vi "Main.vi"() -> ()   [LabVIEW 2021]
doc: "Use this template to build a simple state machine design pattern. Each state executes code and determines which state to transition to."
uses:
  controls/State.ctl
  controls/Data.ctl
  vmmultmso/vmmultmso.lvlib
panel:
  out "Device is OK?":bool
  out "Sample Rate":dbl
  out "Device ID":dbl
  out "CH2 Min":dbl
  out "CH2 Max":dbl
  out "CH2 Vpp":dbl
  out "CH2 Frequency":dbl
  out "CH1 Frequency":dbl
  out "CH1 Vpp":dbl
  out "CH1 Max":dbl
  out "CH1 Min":dbl
  out "IO Read Return":u32 format="%x"
  out "IO4":bool
  out "IO0":bool
  out "Is IO Ready?":bool
  in  "DDS2 Amplitude":dbl=2000.0
  in  "DDS2 Bias":dbl
  in  "DDS2 Freq":dbl=1000.0
  in  "DDS2 Wave Style":u16(ring) items=["Sine", "Square", "Ramp"]
  in  "DDS1 Amplitude":dbl=2000.0
  in  "DDS1 Bias":dbl
  in  "DDS1 Freq":dbl=1000.0
  in  "DDS1 Wave Style":u16(ring) items=["Sine", "Square", "Ramp"]
  out "Is Data Ready？":bool
  out "ReadVoltageData Return":u32
  out "Voltage Wave":dbl[][](graph)
  out "Capture Return":i32
  out "Support Samples":u32[](array[numeric])
  in  "Exit":bool
  # "DDS1"
  # "DDS2"
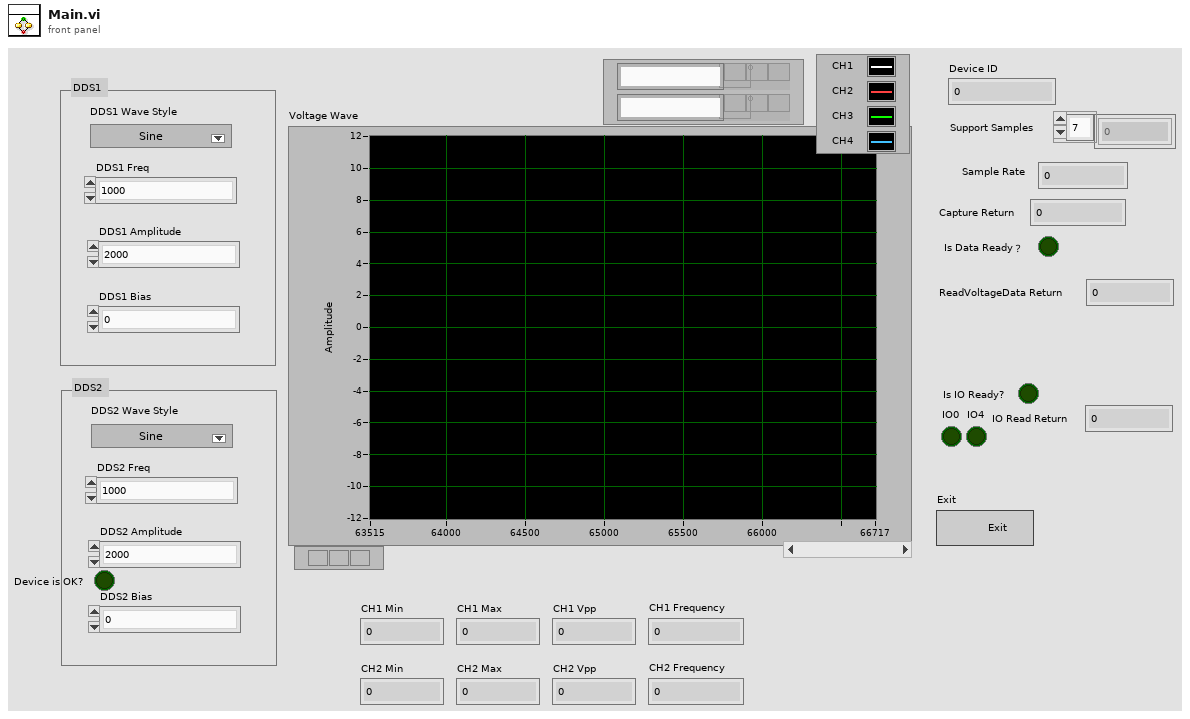
[diagram p1: front panel]
types:
  T1 = typedef "Data.ctl" = cluster{"Boolean <Is Exit>":bool, "String <Replace Me>":string, "Captue Length":dbl, "Device ID":dbl}
  T2 = typedef "State.ctl" = enum16{"Initialize", "Wait for UsbIn", "Init Osc and Dds", "Wait for Event", "Capture", "Read Voltage", "Read IO", "Exit"}
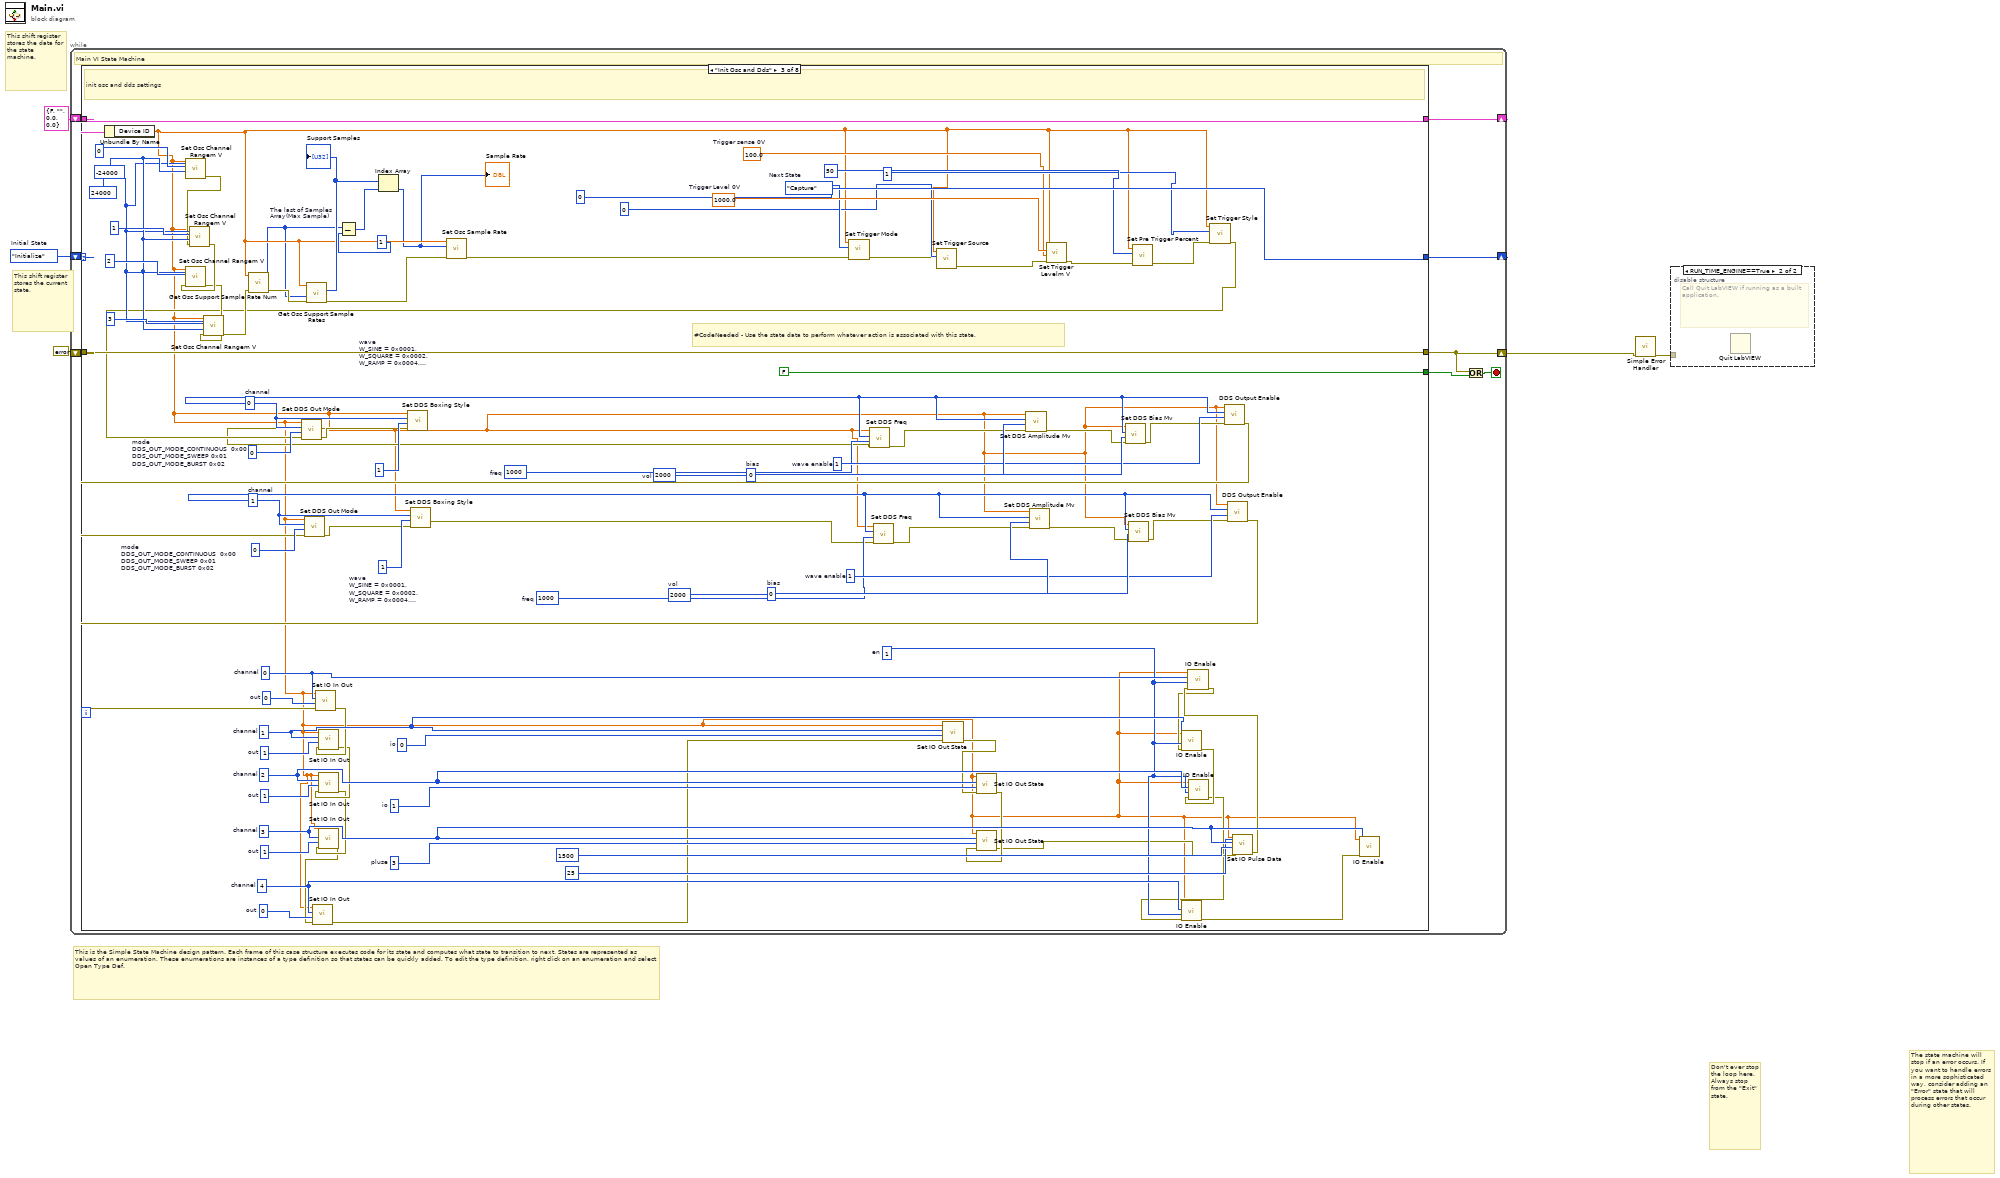
[diagram p0: block diagram]
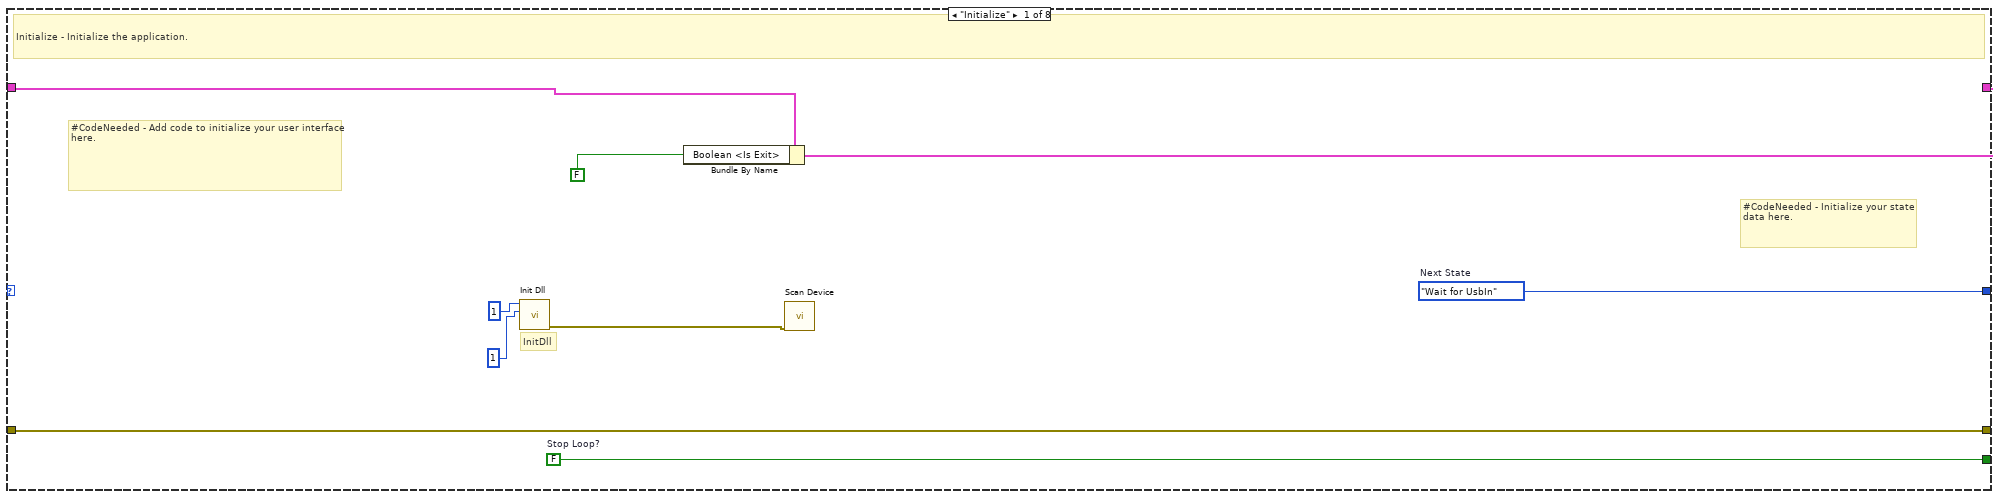
[diagram p3: hidden frame]
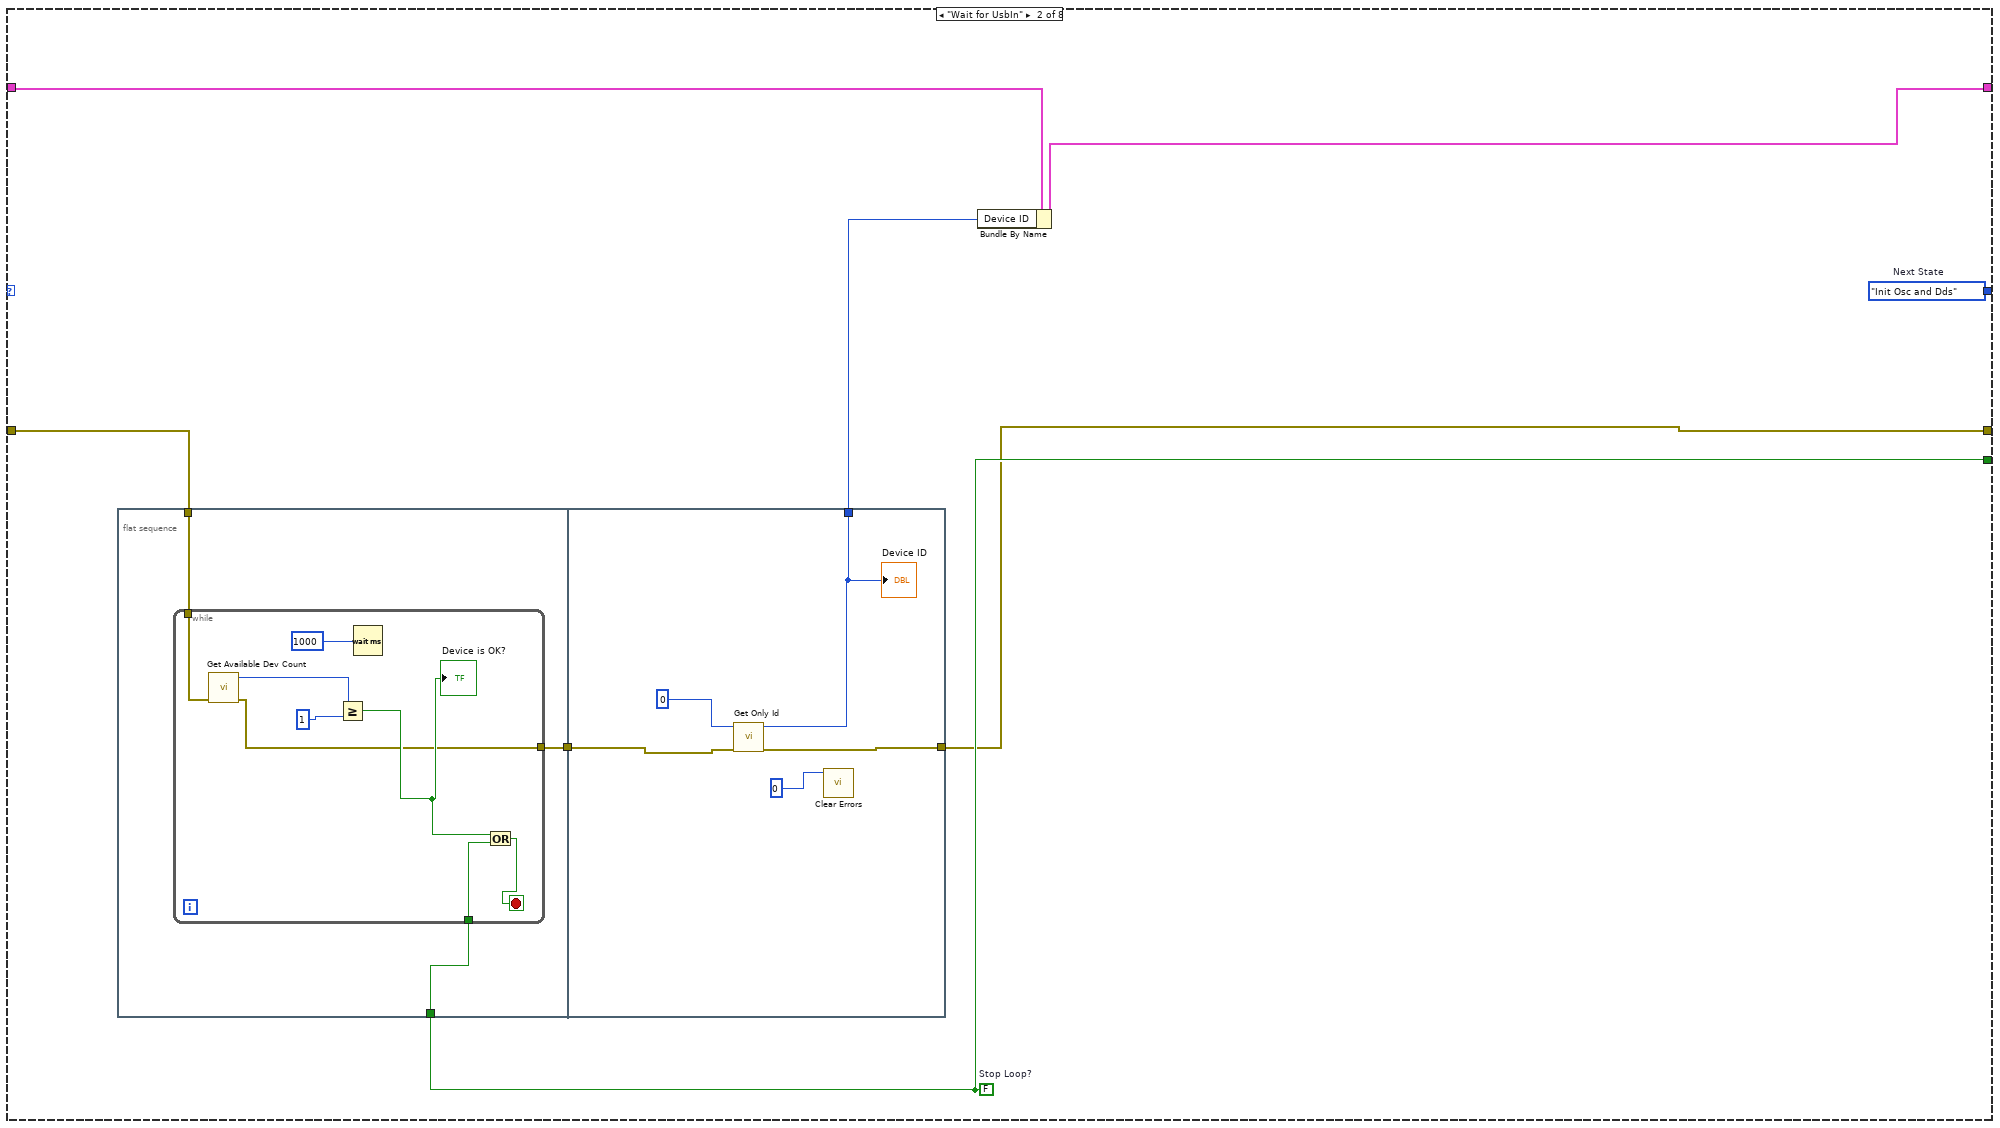
[diagram p4: hidden frame]
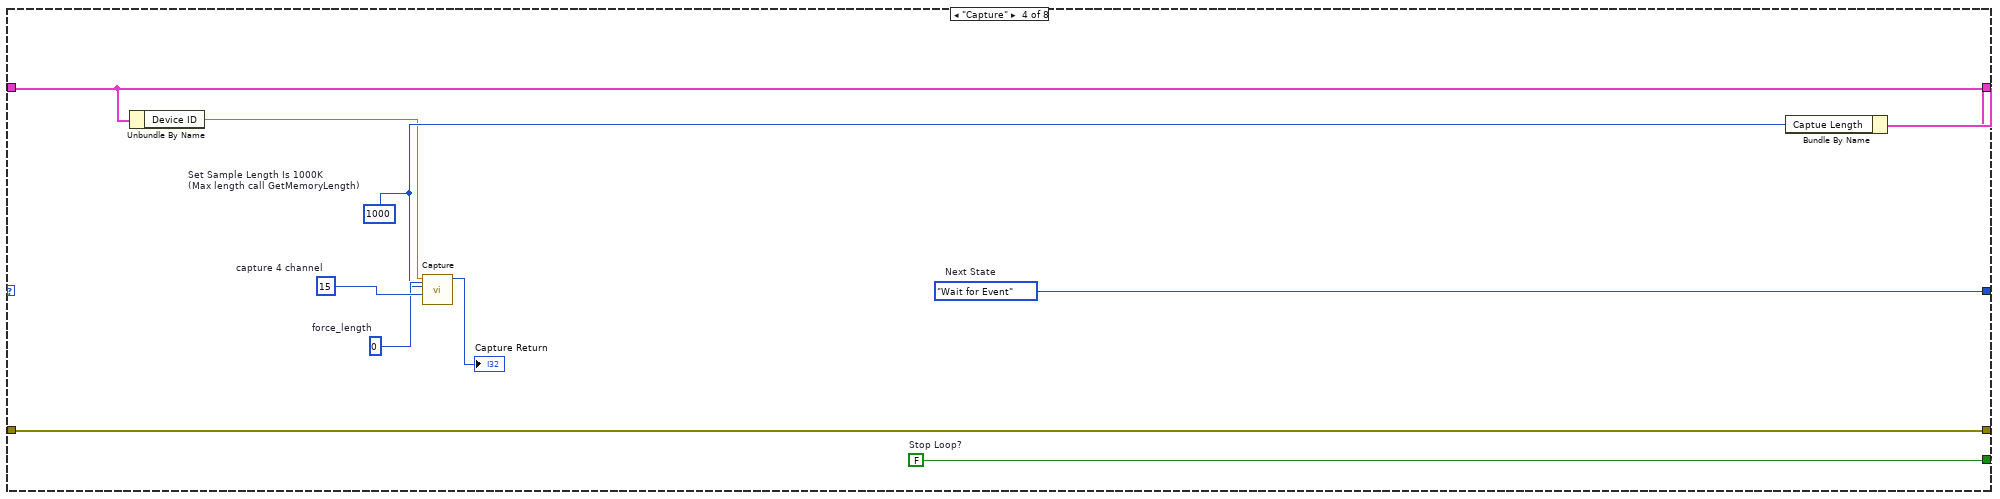
[diagram p5: hidden frame]
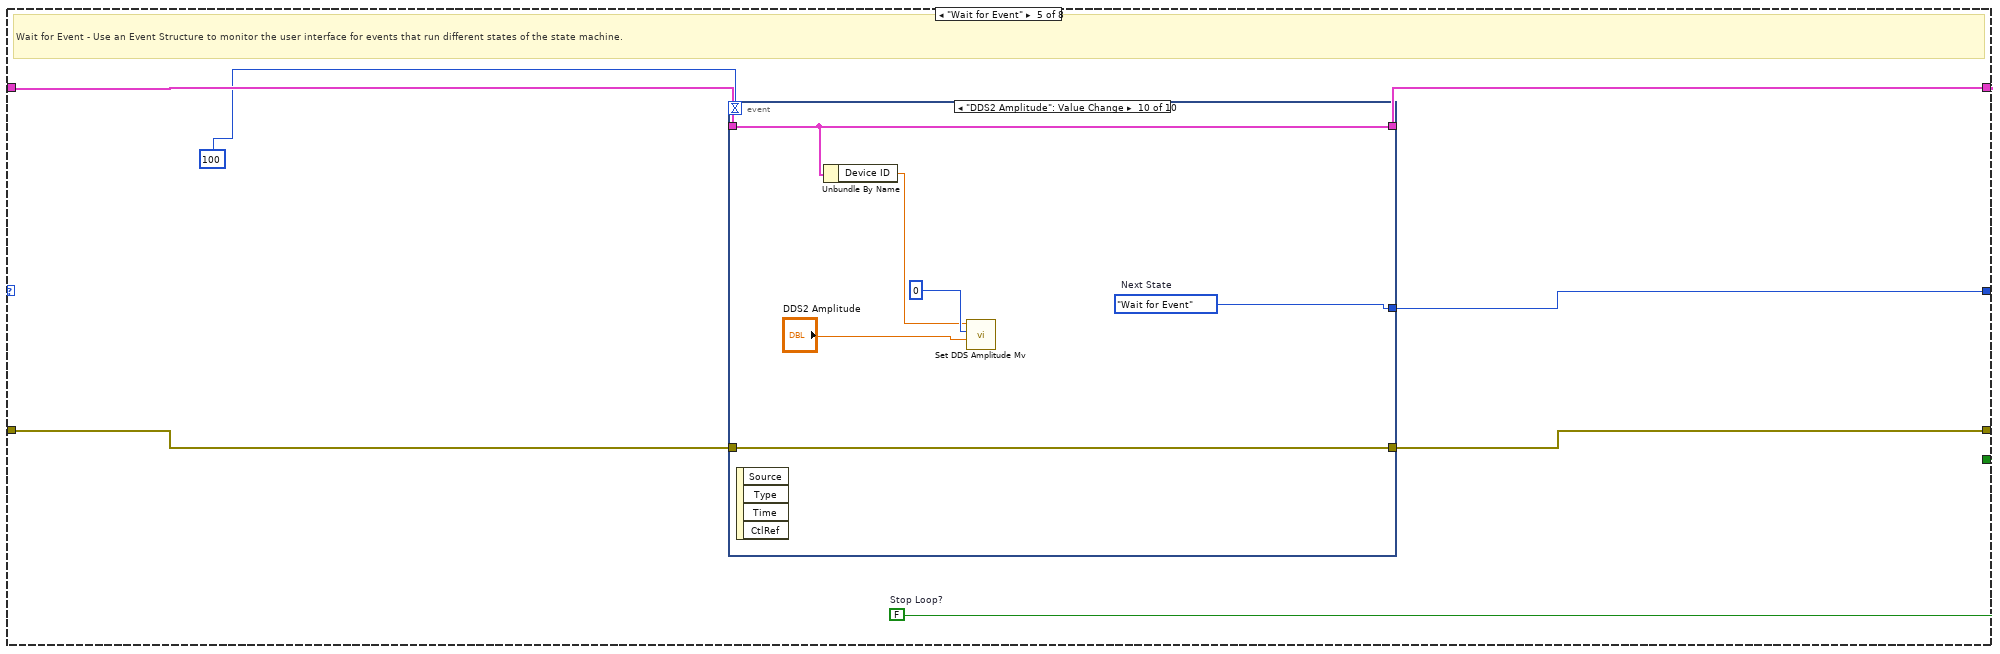
[diagram p6: hidden frame]
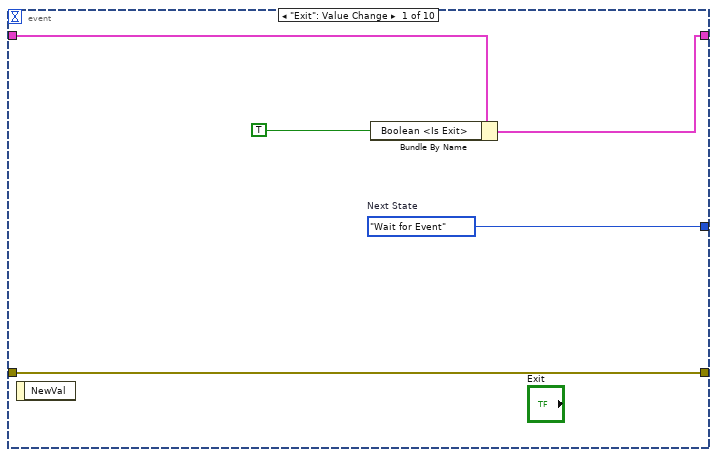
[diagram p7: hidden frame]
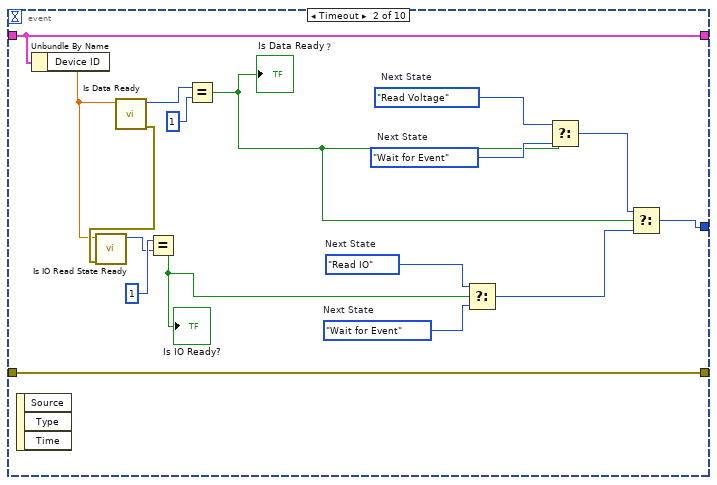
[diagram p8: hidden frame]
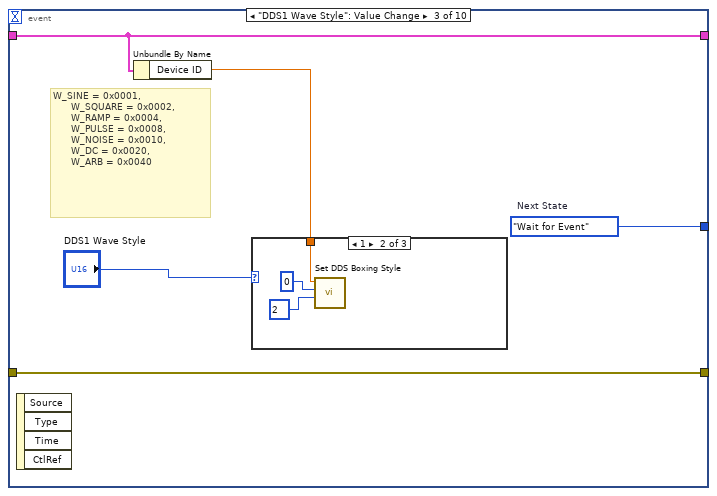
[diagram p9: hidden frame]
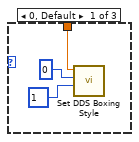
[diagram p10: hidden frame]
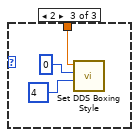
[diagram p11: hidden frame]
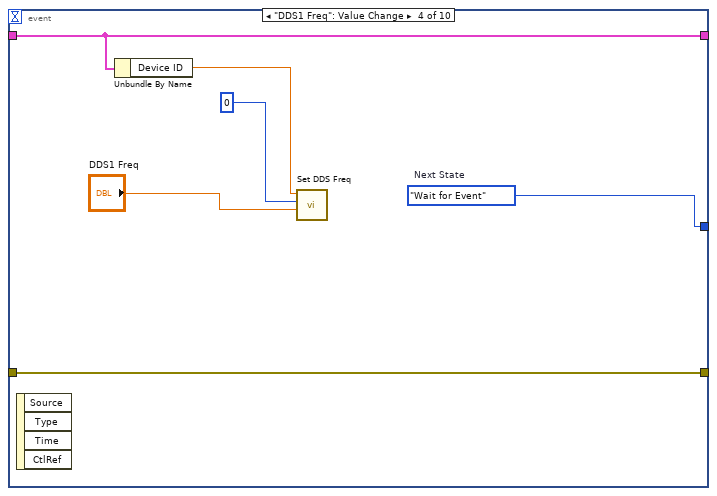
[diagram p12: hidden frame]
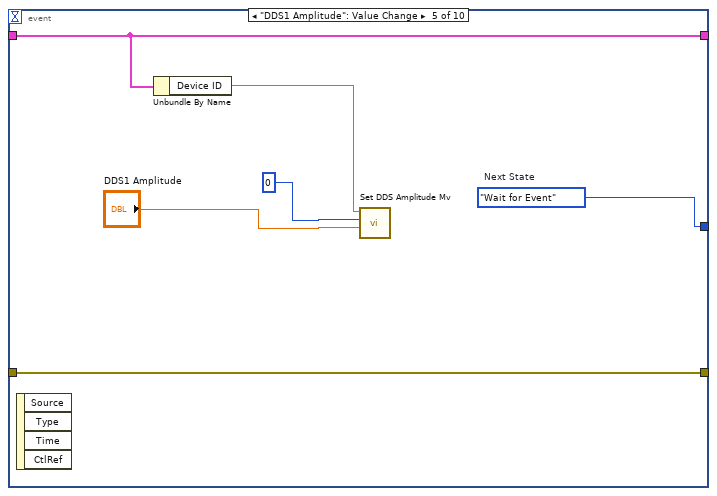
[diagram p13: hidden frame]
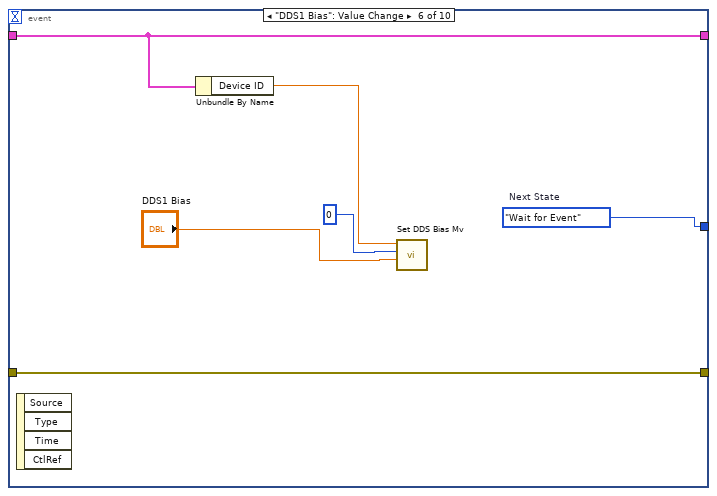
[diagram p14: hidden frame]
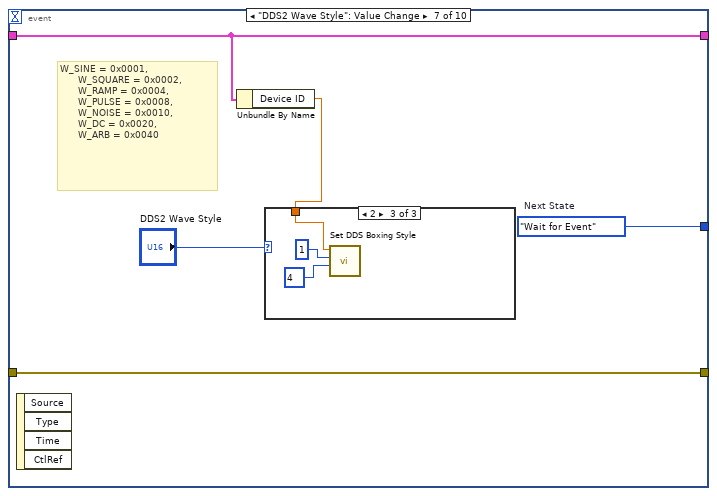
[diagram p15: hidden frame]
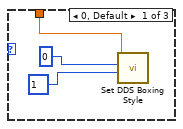
[diagram p16: hidden frame]
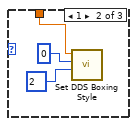
[diagram p17: hidden frame]
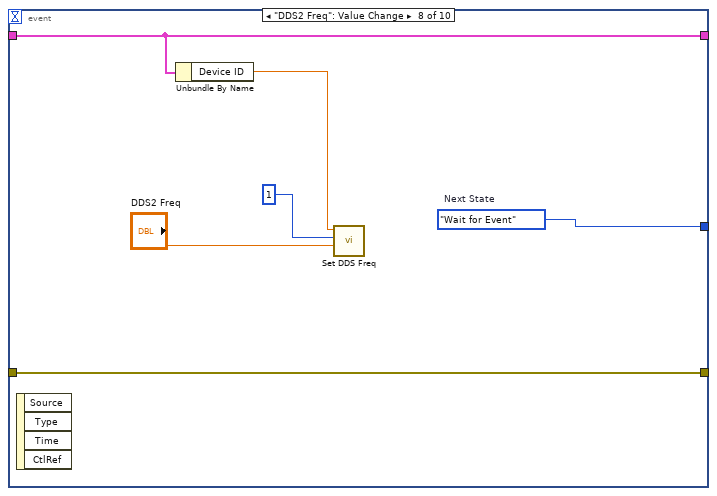
[diagram p18: hidden frame]
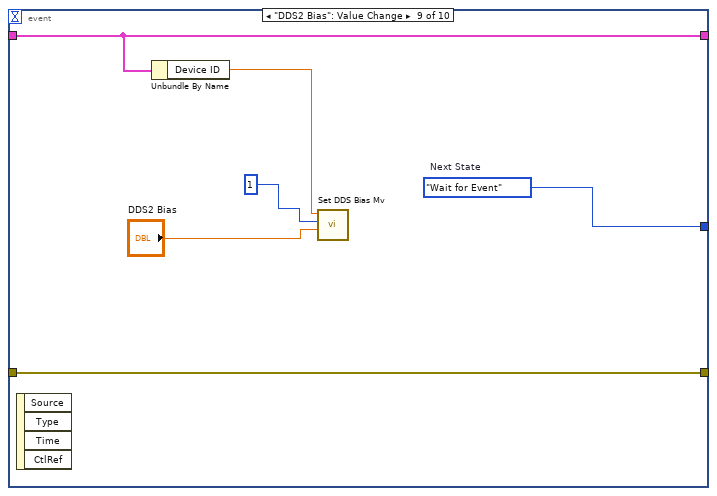
[diagram p19: hidden frame]
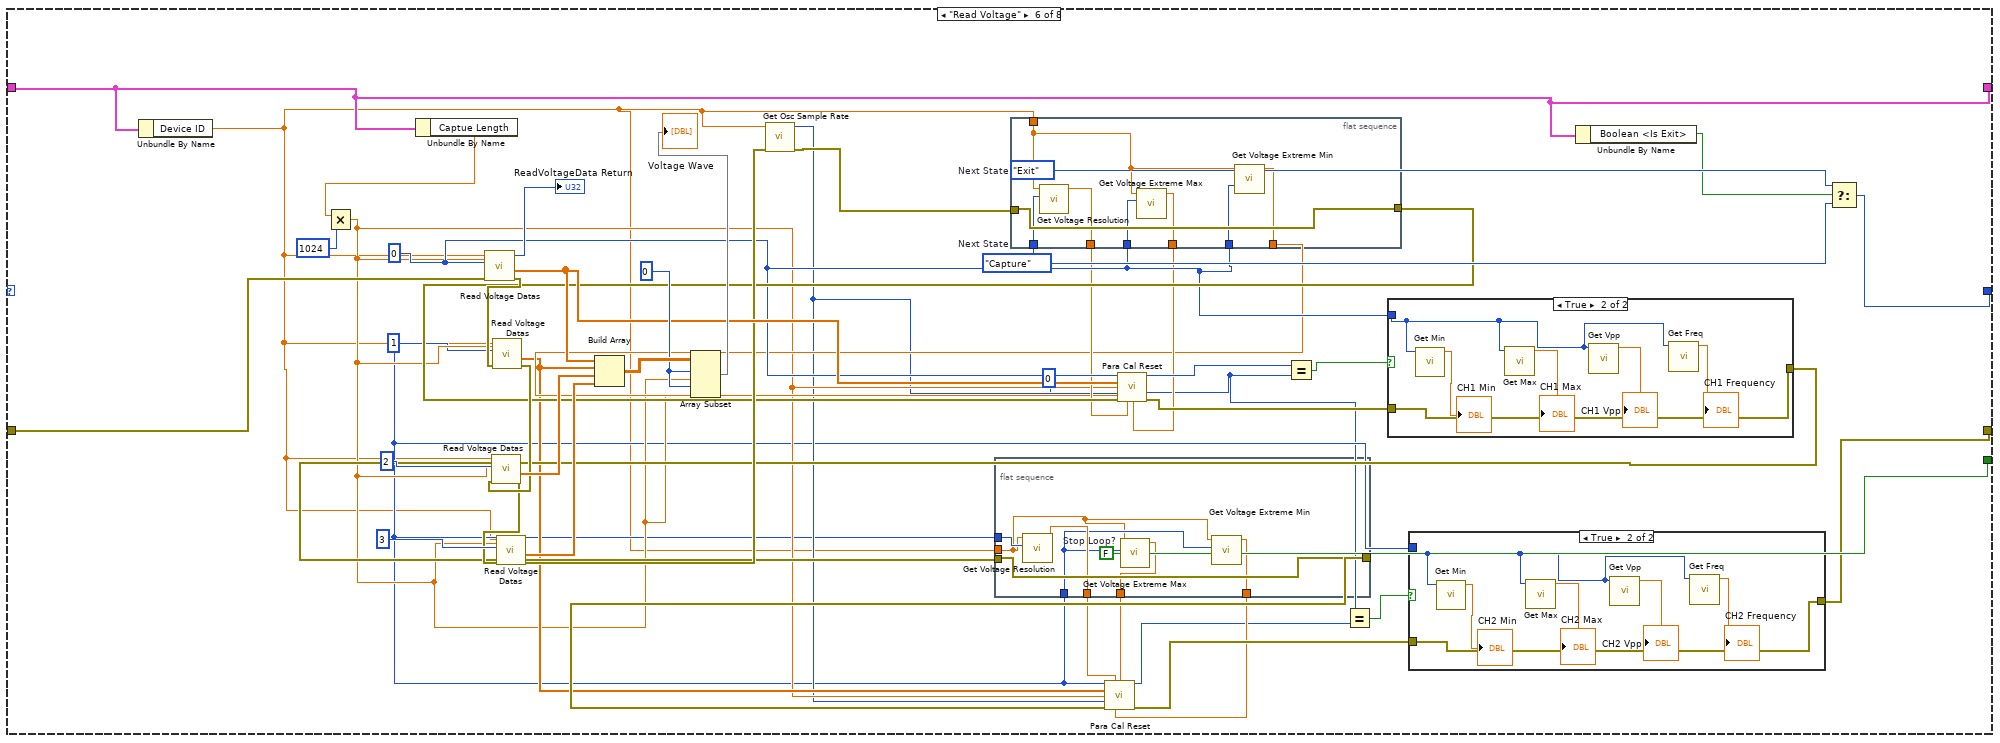
[diagram p20: hidden frame]
diagram:
  w5 = State."Initialize"  # Initial State
  # "Don't ever stop the loop here. Always stop from the \"Exit\" state."
  # "The state machine will stop if an error occurs. If you want to handle errors in a more sophisticated way, consider adding an \"Error\" state that will process errors that occur during other states."
  # "This shift register stores the data for the state machine."
  # "This is the Simple State Machine design pattern. Each frame of this case structure executes code for its state and computes what state to transition to next. States are represented as values of an enumeration. These enumerations are instances of a type definition so that states can be quickly added. To edit the type definition, right click on an enumeration and select Open Type Def."
  # "This shift register stores the current state."
  n1 = while {
    shift-right: [w12] -> _
    shift-left: w5 -> [w13]
    shift-right: [w10] -> _
    shift-left: T1 {"Boolean <Is Exit>"=FALSE, "String <Replace Me>"="", "Captue Length"=0.0, "Device ID"=0.0} ("Data") -> [w11]
    shift-right: [w7] -> w2
    shift-left: errorcluster {"status"=FALSE, "code"=0, "source"=""} ("error constant") -> [w9]
    stop <- w8 stop-if-true
    # "Main VI State Machine"
    n2 = case shown="\"Init Osc and Dds\"" w13 {
      tunnel: [w22 w30 w135 w144 w152 w268 w317 w332] -> w12
      tunnel: w11 -> [w14 w29 w51 w137 w151 w240 w315 w328]
      tunnel: [w15 w28 w51 w139 w150 w240 w315 w328] -> w10
      tunnel: w9 -> [w20 w23 w133 w145 w149 w262 w325 w330]
      tunnel: [w20 w24 w133 w145 w148 w253 w325 w330] -> w7
      tunnel: [w21 w27 FALSE ("Stop Loop?") w143 w146 w284 w316 w331] -> w6
      frame "Initialize" {
        w21 = FALSE  # Stop Loop?
        w22 = State."Wait for UsbIn"  # Next State
        # "InitDll"
        # "#CodeNeeded - Initialize your state data here."
        # "#CodeNeeded - Add code to initialize your user interface here."
        # "Initialize - Initialize the application."
        n3 = call "Init Dll.vi"("en_hard_watchdog"=1 ("channel"), "en_log"=1 ("channel")) -> ("error out"=w17:errorcluster)  [unwired: 8 in, 1 out]
        n4 = Bundle By Name(cluster=w14, "Boolean <Is Exit>"=FALSE) -> (w15:T1)
        n5 = call "Scan Device.vi"("error in (no error)"=w17) -> ()  [unwired: 9 in, 2 out]
      }
      frame "Wait for UsbIn" {
        w27 = FALSE  # Stop Loop?
        w30 = State."Init Osc and Dds"  # Next State
        n6 = flat-sequence {
          tunnel: w27 -> [w33]
          tunnel: [w32] -> w25
          tunnel: w23 -> [w31]
          tunnel: [w45] -> w26
          tunnel: w25 -> [w44]
          tunnel: [w42] -> w24
          frame #0 {
            n7 = while {
              tunnel: w33 -> [w40]
              tunnel: [w35] -> w32
              tunnel: w31 -> [w34]
              stop <- w39 stop-if-true
              n8 = call "Get Available Dev Count.vi"("error in (no error)"=w34) -> ("error out"=w35:errorcluster, "function return"=w38:i32)  [unwired: 9 in]
              n9 = Greater Or Equal?(x=w38, y=1 ("channel")) -> (x >= y?=w36:bool)
              "Device is OK?" <- w36
              n10 = Wait (ms)(milliseconds to wait=u32 1000 ("等待时间（毫秒）")) -> ()  [unwired: 1 out]
              n11 = Or(x=w36, y=w40) -> (x .or. y?=w39:bool)
            }
          }
          frame #1 {
            n12 = call "Get Only Id.vi"("error in (no error)"=w44, "dev_index"=0 ("channel")) -> ("error out"=w42:errorcluster, "function return"=w45:u32)  [unwired: 8 in]
            "Device ID" <- w45
            n13 = call <vilib>:"Clear Errors.vi"("specific error code to clear (0: all)"=0 ("channel")) -> ()  [unwired: 5 in, 2 out]
          }
        }
        n14 = Bundle By Name(cluster=w29, "Device ID"=w26) -> (w28:T1)
      }
      frame "Init Osc and Dds" {
        w95 = i8 0  # out
        w94 = i8 4  # channel
        w99 = i8 3  # pluse
        w100 = i8 1  # out
        w98 = i8 3  # channel
        w93 = i8 1  # en
        w104 = i8 0  # io
        w105 = i8 1  # io
        w106 = i8 1  # out
        w101 = i8 2  # channel
        w107 = i8 1  # out
        w102 = i8 1  # channel
        w108 = i8 0  # out
        w103 = i8 0  # channel
        w109 = sgl 100.0  # Trigger sense 0V
        w115 = i8 0  # mode DDS_OUT_MODE_CONTINUOUS  0x00 DDS_OUT_MODE_SWEEP 0x01 DDS_OUT_MODE_BURST 0x02
        w116 = i8 1  # wave enable
        w118 = u32 0  # bias
        w117 = u32 2000  # vol
        w54 = u32 1000  # freq
        w119 = i8 1  # wave  W_SINE = 0x0001,  W_SQUARE = 0x0002,  W_RAMP = 0x0004,  W_PULSE = 0x0008,  W_NOISE = 0x0010,  W_DC = 0x0020,  W_ARB = 0x0040
        w55 = i8 1  # channel
        w120 = i8 0  # mode DDS_OUT_MODE_CONTINUOUS  0x00 DDS_OUT_MODE_SWEEP 0x01 DDS_OUT_MODE_BURST 0x02
        w121 = i8 1  # wave enable
        w123 = u32 0  # bias
        w122 = u32 2000  # vol
        w58 = u32 1000  # freq
        w124 = i8 1  # wave  W_SINE = 0x0001,  W_SQUARE = 0x0002,  W_RAMP = 0x0004,  W_PULSE = 0x0008,  W_NOISE = 0x0010,  W_DC = 0x0020,  W_ARB = 0x0040
        w59 = i8 0  # channel
        w130 = sgl 1000.0  # Trigger Level 0V
        w110 = 24000 ("minmv")
        w111 = -24000 ("minmv")
        w135 = State."Capture"  # Next State
        # "#CodeNeeded - Use the state data to perform whatever action is associated with this state."
        # "init osc and dds settings"
        n15 = Unbundle By Name(w51) -> ("Device ID"=w50:dbl)
        n16 = call "Set Osc Channel Rangem V.vi"("maxmv"=w110, "minmv"=w111, "channel"=0, "dev_id"=w50) -> ("error out"=w92:errorcluster)  [unwired: 6 in, 1 out]
        n17 = call "Set Osc Channel Rangem V.vi"("maxmv"=w110, "error in (no error)"=w92, "minmv"=w111, "channel"=1, "dev_id"=w50) -> ("error out"=w91:errorcluster)  [unwired: 5 in, 1 out]
        n18 = call "Set Osc Channel Rangem V.vi"("maxmv"=w110, "error in (no error)"=w91, "minmv"=w111, "channel"=2, "dev_id"=w50) -> ("error out"=w90:errorcluster)  [unwired: 5 in, 1 out]
        n19 = call "Set Osc Channel Rangem V.vi"("maxmv"=w110, "error in (no error)"=w90, "minmv"=w111, "channel"=3, "dev_id"=w50) -> ("error out"=w89:errorcluster)  [unwired: 5 in, 1 out]
        n20 = call "Get Osc Support Sample Rate Num.vi"("error in (no error)"=w89, "dev_id"=w50) -> ("error out"=w88:errorcluster, "function return"=w48:i32)  [unwired: 8 in]
        n21 = call "Get Osc Support Sample Rates.vi"("error in (no error)"=w88, "maxnum"=w48, "dev_id"=w50) -> ("error out"=w87:errorcluster, "sample out"=w126:u32[])  [unwired: 6 in, 1 out]
        "Support Samples" <- w126
        n22 = Subtract "The last of Samples Array(Max Sample)"(x=w48, y=1 ("front")) -> (x-y=w47:i32)
        n23 = Index Array(array=w126, index=w47) -> (element=w49:u32)
        "Sample Rate" <- w49
        n24 = call "Set Osc Sample Rate.vi"("error in (no error)"=w87, "sample"=w49, "dev_id"=w50) -> ("error out"=w86:errorcluster)  [unwired: 7 in, 1 out]
        n25 = call "Set Trigger Mode.vi"("error in (no error)"=w86, "mode"=0 ("front"), "dev_id"=w50) -> ("error out"=w85:errorcluster)  [unwired: 8 in]
        n26 = call "Set Trigger Source.vi"("error in (no error)"=w85, "source"=0 ("front"), "dev_id"=w50) -> ("error out"=w84:errorcluster)  [unwired: 8 in]
        n27 = call "Set Trigger Levelm V.vi"("error in (no error)"=w84, "sense_mv"=w109, "level_mv"=w130, "dev_id"=w50) -> ("error out"=w83:errorcluster)  [unwired: 7 in]
        n28 = call "Set Pre Trigger Percent.vi"("error in (no error)"=w83, "front"=50, "dev_id"=w50) -> ("error out"=w82:errorcluster)  [unwired: 8 in]
        n29 = call "Set Trigger Style.vi"("error in (no error)"=w82, "style"=u32 1, "dev_id"=w50) -> ("error out"=w81:errorcluster)  [unwired: 8 in]
        n30 = call "Set DDS Out Mode.vi"("error in (no error)"=w81, "out_mode"=w120, "channel_index"=w59, "dev_id"=w50) -> ("error out"=w80:errorcluster)  [unwired: 7 in]
        n31 = call "Set DDS Boxing Style.vi"("error in (no error)"=w80, "boxing"=w124, "channel_index"=w59, "dev_id"=w50) -> ("error out"=w57:errorcluster)  [unwired: 7 in]
        n32 = call "Set DDS Freq.vi"("error in (no error)"=w57, "freq"=w58, "channel_index"=w59, "dev_id"=w50) -> ("error out"=w56:errorcluster)  [unwired: 7 in]
        n33 = call "Set DDS Amplitude Mv.vi"("error in (no error)"=w56, "amplitdude"=w122, "channel_index"=w59, "dev_id"=w50) -> ("error out"=w79:errorcluster)  [unwired: 7 in]
        n34 = call "Set DDS Bias Mv.vi"("error in (no error)"=w79, "bias"=w123, "channel_index"=w59, "dev_id"=w50) -> ("error out"=w78:errorcluster)  [unwired: 7 in]
        n35 = call "DDS Output Enable.vi"("error in (no error)"=w78, "enable"=w121, "channel_index"=w59, "dev_id"=w50) -> ("error out"=w77:errorcluster)  [unwired: 7 in]
        n36 = call "Set DDS Out Mode.vi"("error in (no error)"=w77, "out_mode"=w115, "channel_index"=w55, "dev_id"=w50) -> ("error out"=w76:errorcluster)  [unwired: 7 in]
        n37 = call "Set DDS Boxing Style.vi"("error in (no error)"=w76, "boxing"=w119, "channel_index"=w55, "dev_id"=w50) -> ("error out"=w53:errorcluster)  [unwired: 7 in]
        n38 = call "Set DDS Freq.vi"("error in (no error)"=w53, "freq"=w54, "channel_index"=w55, "dev_id"=w50) -> ("error out"=w52:errorcluster)  [unwired: 7 in]
        n39 = call "Set DDS Amplitude Mv.vi"("error in (no error)"=w52, "amplitdude"=w117, "channel_index"=w55, "dev_id"=w50) -> ("error out"=w75:errorcluster)  [unwired: 7 in]
        n40 = call "Set DDS Bias Mv.vi"("error in (no error)"=w75, "bias"=w118, "channel_index"=w55, "dev_id"=w50) -> ("error out"=w74:errorcluster)  [unwired: 7 in]
        n41 = call "DDS Output Enable.vi"("error in (no error)"=w74, "enable"=w116, "channel_index"=w55, "dev_id"=w50) -> ("error out"=w73:errorcluster)  [unwired: 7 in]
        n42 = call "Set IO In Out.vi"("error in (no error)"=w73, "inout"=w108, "channel"=w103, "dev_id"=w50) -> ("error out"=w72:errorcluster)  [unwired: 7 in]
        n43 = call "Set IO In Out.vi"("error in (no error)"=w72, "inout"=w107, "channel"=w102, "dev_id"=w50) -> ("error out"=w71:errorcluster)  [unwired: 7 in]
        n44 = call "Set IO In Out.vi"("error in (no error)"=w71, "inout"=w106, "channel"=w101, "dev_id"=w50) -> ("error out"=w70:errorcluster)  [unwired: 7 in]
        n45 = call "Set IO In Out.vi"("error in (no error)"=w70, "inout"=w100, "channel"=w98, "dev_id"=w50) -> ("error out"=w69:errorcluster)  [unwired: 7 in]
        n46 = call "Set IO In Out.vi"("error in (no error)"=w69, "inout"=w95, "channel"=w94, "dev_id"=w50) -> ("error out"=w68:errorcluster)  [unwired: 7 in]
        n47 = call "Set IO Out State.vi"("error in (no error)"=w68, "state"=w104, "channel"=w102, "dev_id"=w50) -> ("error out"=w67:errorcluster)  [unwired: 7 in]
        n48 = call "Set IO Out State.vi"("error in (no error)"=w67, "state"=w105, "channel"=w101, "dev_id"=w50) -> ("error out"=w66:errorcluster)  [unwired: 7 in]
        n49 = call "Set IO Out State.vi"("error in (no error)"=w66, "state"=w99, "channel"=w98, "dev_id"=w50) -> ("error out"=w65:errorcluster)  [unwired: 7 in]
        n50 = call "Set IO Pulse Data.vi"("duty"=25 ("minmv"), "error in (no error)"=w65, "hz"=1500 ("minmv"), "channel"=w98, "dev_id"=w50) -> ("error out"=w64:errorcluster)  [unwired: 6 in]
        n51 = call "IO Enable.vi"("error in (no error)"=w64, "enable"=w93, "channel"=w103, "dev_id"=w50) -> ("error out"=w63:errorcluster)  [unwired: 7 in]
        n52 = call "IO Enable.vi"("error in (no error)"=w63, "enable"=w93, "channel"=w102, "dev_id"=w50) -> ("error out"=w62:errorcluster)  [unwired: 7 in]
        n53 = call "IO Enable.vi"("error in (no error)"=w62, "enable"=w93, "channel"=w101, "dev_id"=w50) -> ("error out"=w61:errorcluster)  [unwired: 7 in]
        n54 = call "IO Enable.vi"("error in (no error)"=w61, "enable"=w93, "channel"=w94, "dev_id"=w50) -> ("error out"=w60:errorcluster)  [unwired: 7 in]
        n55 = call "IO Enable.vi"("error in (no error)"=w60, "channel"=w98, "dev_id"=w50) -> ()  [unwired: 8 in, 1 out]
      }
      frame "Capture" {
        w140 = i8 0  # force_length
        w138 = u32 1000  # Set Sample Length Is 1000K (Max length call GetMemoryLength)
        w141 = i8 15  # capture 4 channel
        w143 = FALSE  # Stop Loop?
        w144 = State."Wait for Event"  # Next State
        n56 = Unbundle By Name(w137) -> ("Device ID"=w136:dbl)
        n57 = call "Capture.vi"("force_length"=w140, "capture_channel"=w141, "length"=w138, "dev_id"=w136) -> ("function return"=→"Capture Return":i32)  [unwired: 6 in, 1 out]
        n58 = Bundle By Name(cluster=w137, "Captue Length"=w138) -> (w139:T1)
      }
      frame "Wait for Event" {
        w146 = FALSE  # Stop Loop?
        # "Wait for Event - Use an Event Structure to monitor the user interface for events that run different states of the state machine."
        n59 = event shown="[9] \"DDS2 Amplitude\": Value Change" {
          selector: _ -> [_ _ _ _ _ _ _ _ _ _]
          dyn-events: _ -> [_ _ _ _ _ _ _ _ _ _]
          timeout: 100 ("y") -> [_ _ _ _ _ _ _ _ _ _]
          tunnel: [w157 w162 w177 w193 w199 w205 w210 w225 w230 w236] -> w152
          tunnel: w151 -> [w154 w159 w176 w189 w196 w202 w208 w222 w228 w233]
          tunnel: [w153 w159 w176 w189 w196 w202 w208 w222 w228 w233] -> w150
          tunnel: w149 -> [w156 w174 w179 w194 w200 w206 w211 w226 w232 w238]
          tunnel: [w156 w174 w179 w194 w200 w206 w211 w226 w232 w238] -> w148
          event "Exit": Value Change {
            w157 = State."Wait for Event"  # Next State
            n60 = event-data() -> ()  [unwired: 1 in, 1 out]
            n61 = Bundle By Name(cluster=w154, "Boolean <Is Exit>"=TRUE) -> (w153:T1)
          }
          event Timeout {
            w167 = State."Wait for Event"  # Next State
            w168 = State."Read IO"  # Next State
            w170 = State."Wait for Event"  # Next State
            w171 = State."Read Voltage"  # Next State
            n62 = event-data() -> ()  [unwired: 1 in, 3 out]
            n63 = Unbundle By Name(w159) -> ("Device ID"=w158:dbl)
            n64 = call "Is Data Ready.vi"("dev_id"=w158) -> ("error out"=w160:errorcluster, "function return"=w173:i32)  [unwired: 9 in]
            n65 = call "Is IO Read State Ready.vi"("error in (no error)"=w160, "dev_id"=w158) -> ("function return"=w161:i32)  [unwired: 8 in, 1 out]
            n66 = Equal?(x=1 ("y"), y=w161) -> (x = y?=w169:bool)
            "Is IO Ready?" <- w169
            n67 = Equal?(x=w173, y=1) -> (x = y?=w163:bool)
            "Is Data Ready？" <- w163
            n68 = Select(t=w168, s=w169, f=w167) -> (s? t:f=w165:T2)
            n69 = Select(t=w171, s=w163, f=w170) -> (s? t:f=w164:T2)
            n70 = Select(t=w164, s=w163, f=w165) -> (s? t:f=w162:T2)
          }
          event "DDS1 Wave Style": Value Change {
            w177 = State."Wait for Event"  # Next State
            # "W_SINE = 0x0001, \n\t\t\t\t\t\tW_SQUARE = 0x0002, \n\t\t\t\t\t\tW_RAMP = 0x0004, \n\t\t\t\t\t\tW_PULSE = 0x0008, \n\t\t\t\t\t\tW_NOISE = 0x0010, \n\t\t\t\t\t\tW_DC = 0x0020, \n\t\t\t\t\t\tW_ARB = 0x0040"
            n71 = event-data() -> ()  [unwired: 1 in, 4 out]
            n72 = Unbundle By Name(w176) -> ("Device ID"=w175:dbl)
            n73 = case shown="1" "DDS1 Wave Style" {
              tunnel: w175 -> [w180 w183 w186]
              frame 0, Default {
                n74 = call "Set DDS Boxing Style.vi"("boxing"=1 ("y"), "channel_index"=0 ("y"), "dev_id"=w180) -> ()  [unwired: 8 in, 1 out]
              }
              frame 1 {
                n75 = call "Set DDS Boxing Style.vi"("boxing"=2 ("y"), "channel_index"=0 ("y"), "dev_id"=w183) -> ()  [unwired: 8 in, 1 out]
              }
              frame 2 {
                n76 = call "Set DDS Boxing Style.vi"("boxing"=4 ("y"), "channel_index"=0 ("y"), "dev_id"=w186) -> ()  [unwired: 8 in, 1 out]
              }
            }
          }
          event "DDS1 Freq": Value Change {
            w193 = State."Wait for Event"  # Next State
            n77 = event-data() -> ()  [unwired: 1 in, 4 out]
            n78 = Unbundle By Name(w189) -> ("Device ID"=w190:dbl)
            n79 = call "Set DDS Freq.vi"("freq"="DDS1 Freq", "channel_index"=0 ("y"), "dev_id"=w190) -> ()  [unwired: 8 in, 1 out]
          }
          event "DDS1 Amplitude": Value Change {
            w199 = State."Wait for Event"  # Next State
            n80 = event-data() -> ()  [unwired: 1 in, 4 out]
            n81 = Unbundle By Name(w196) -> ("Device ID"=w195:dbl)
            n82 = call "Set DDS Amplitude Mv.vi"("amplitdude"="DDS1 Amplitude", "channel_index"=0 ("y"), "dev_id"=w195) -> ()  [unwired: 8 in, 1 out]
          }
          event "DDS1 Bias": Value Change {
            w205 = State."Wait for Event"  # Next State
            n83 = event-data() -> ()  [unwired: 1 in, 4 out]
            n84 = Unbundle By Name(w202) -> ("Device ID"=w201:dbl)
            n85 = call "Set DDS Bias Mv.vi"("bias"="DDS1 Bias", "channel_index"=0 ("y"), "dev_id"=w201) -> ()  [unwired: 8 in, 1 out]
          }
          event "DDS2 Wave Style": Value Change {
            w210 = State."Wait for Event"  # Next State
            # "W_SINE = 0x0001, \n\t\t\t\t\t\tW_SQUARE = 0x0002, \n\t\t\t\t\t\tW_RAMP = 0x0004, \n\t\t\t\t\t\tW_PULSE = 0x0008, \n\t\t\t\t\t\tW_NOISE = 0x0010, \n\t\t\t\t\t\tW_DC = 0x0020, \n\t\t\t\t\t\tW_ARB = 0x0040"
            n86 = event-data() -> ()  [unwired: 1 in, 4 out]
            n87 = Unbundle By Name(w208) -> ("Device ID"=w207:dbl)
            n88 = case shown="2" "DDS2 Wave Style" {
              tunnel: w207 -> [w212 w215 w218]
              frame 0, Default {
                n89 = call "Set DDS Boxing Style.vi"("boxing"=1 ("y"), "channel_index"=0 ("y"), "dev_id"=w212) -> ()  [unwired: 8 in, 1 out]
              }
              frame 1 {
                n90 = call "Set DDS Boxing Style.vi"("boxing"=2 ("y"), "channel_index"=0 ("y"), "dev_id"=w215) -> ()  [unwired: 8 in, 1 out]
              }
              frame 2 {
                n91 = call "Set DDS Boxing Style.vi"("boxing"=4 ("y"), "channel_index"=1 ("y"), "dev_id"=w218) -> ()  [unwired: 8 in, 1 out]
              }
            }
          }
          event "DDS2 Freq": Value Change {
            w225 = State."Wait for Event"  # Next State
            n92 = event-data() -> ()  [unwired: 1 in, 4 out]
            n93 = Unbundle By Name(w222) -> ("Device ID"=w221:dbl)
            n94 = call "Set DDS Freq.vi"("freq"="DDS2 Freq", "channel_index"=1 ("y"), "dev_id"=w221) -> ()  [unwired: 8 in, 1 out]
          }
          event "DDS2 Bias": Value Change {
            w230 = State."Wait for Event"  # Next State
            n95 = event-data() -> ()  [unwired: 1 in, 4 out]
            n96 = Unbundle By Name(w228) -> ("Device ID"=w227:dbl)
            n97 = call "Set DDS Bias Mv.vi"("bias"="DDS2 Bias", "channel_index"=1 ("y"), "dev_id"=w227) -> ()  [unwired: 8 in, 1 out]
          }
          event "DDS2 Amplitude": Value Change {
            w236 = State."Wait for Event"  # Next State
            n98 = event-data() -> ()  [unwired: 1 in, 4 out]
            n99 = Unbundle By Name(w233) -> ("Device ID"=w234:dbl)
            n100 = call "Set DDS Amplitude Mv.vi"("amplitdude"="DDS2 Amplitude", "channel_index"=0 ("y"), "dev_id"=w234) -> ()  [unwired: 8 in, 1 out]
          }
        }
      }
      frame "Read Voltage" {
        w241 = i8 0 ("channel")
        w270 = State."Exit"  # Next State
        w269 = State."Capture"  # Next State
        w275 = i8 0 ("channel")
        w244 = i8 1 ("channel")
        w258 = i8 0 ("channel")
        w284 = FALSE  # Stop Loop?
        n101 = Unbundle By Name(w240) -> ("Device ID"=w239:dbl)
        n102 = Unbundle By Name(w240) -> ("Captue Length"=w281:dbl)
        n103 = Multiply(x=w281, y=1024) -> (x*y=w246:dbl)
        n104 = call "Read Voltage Datas.vi"("length"=w246, "error in (no error)"=w262, "channel"=w258, "dev_id"=w239) -> ("error out"=w273:errorcluster, "buffer out"=w266:dbl[], "function return"=→"ReadVoltageData Return":u32)  [unwired: 5 in]
        n105 = call "Read Voltage Datas.vi"("length"=w246, "error in (no error)"=w273, "channel"=w244, "dev_id"=w239) -> ("error out"=w272:errorcluster, "buffer out"=w247:dbl[])  [unwired: 5 in, 1 out]
        n106 = call "Read Voltage Datas.vi"("length"=w246, "error in (no error)"=w272, "channel"=i8 2, "dev_id"=w239) -> ("error out"=w271:errorcluster, "buffer out"=w278:dbl[])  [unwired: 5 in, 1 out]
        n107 = call "Read Voltage Datas.vi"("length"=w246, "error in (no error)"=w271, "channel"=i8 3, "dev_id"=w239) -> ("error out"=w265:errorcluster, "buffer out"=w277:dbl[])  [unwired: 5 in, 1 out]
        n108 = Build Array(w266, w247, w278, w277) -> (w276:dbl[][])
        n109 = Array Subset(array=w276, index (row)=w275, length (row)=w246, index (col)=w275, length (col)=w246) -> (→"Voltage Wave":dbl[][])
        n110 = call "Get Osc Sample Rate.vi"("error in (no error)"=w265, "dev_id"=w239) -> ("error out"=w260:errorcluster, "function return"=w245:u32)  [unwired: 8 in]
        n111 = flat-sequence {
          tunnel: [w298] -> w251
          tunnel: w254 -> [w298]
          tunnel: w244 -> [w294]
          tunnel: w244 -> [w293]
          tunnel: [w297] -> w250
          tunnel: [w296] -> w249
          tunnel: [w295] -> w248
          tunnel: w239 -> [w292]
          frame #0 {
            n112 = call "Get Voltage Resolution.vi"("channel"=w294, "dev_id"=w292) -> ("function return"=w297:dbl)  [unwired: 8 in, 1 out]
            n113 = call "Get Voltage Extreme Max.vi"("channel"=w293, "dev_id"=w292) -> ("function return"=w296:dbl)  [unwired: 8 in, 1 out]
            n114 = call "Get Voltage Extreme Min.vi"("channel"=w293, "dev_id"=w292) -> ("function return"=w295:dbl)  [unwired: 8 in, 1 out]
          }
        }
        n115 = flat-sequence {
          tunnel: [w306] -> w259
          tunnel: w258 -> [w305]
          tunnel: [w304] -> w255
          tunnel: [w303] -> w256
          tunnel: w258 -> [w300]
          tunnel: [w302] -> w257
          tunnel: w258 -> [w301]
          tunnel: w260 -> [w306]
          tunnel: w239 -> [w299]
          frame #0 {
            n116 = call "Get Voltage Resolution.vi"("channel"=w301, "dev_id"=w299) -> ("function return"=w302:dbl)  [unwired: 8 in, 1 out]
            n117 = call "Get Voltage Extreme Max.vi"("channel"=w300, "dev_id"=w299) -> ("function return"=w303:dbl)  [unwired: 8 in, 1 out]
            n118 = call "Get Voltage Extreme Min.vi"("channel"=w305, "dev_id"=w299) -> ("function return"=w304:dbl)  [unwired: 8 in, 1 out]
          }
        }
        n119 = call "Para Cal Reset.vi"("para_chn"=w244, "voltage_resolution"=w250, "extreme_max"=w249, "buffer"=w247, "buffer_length"=w246, "sample"=w245, "error in (no error)"=w251, "extreme_min"=w248) -> ("function return"=w242:i32, "error out"=w252:errorcluster)  [unwired: 5 in, 1 out]
        n120 = call "Para Cal Reset.vi"("para_chn"=w258, "voltage_resolution"=w257, "extreme_max"=w256, "buffer"=w266, "buffer_length"=w246, "sample"=w245, "error in (no error)"=w259, "extreme_min"=w255) -> ("function return"=w263:i32, "error out"=w261:errorcluster)  [unwired: 5 in, 1 out]
        n121 = Equal?(x=w263, y=w241) -> (x = y?=w264:bool)
        n122 = Equal?(x=w241, y=w242) -> (x = y?=w243:bool)
        n123 = case shown="True" w264 {
          tunnel: w258 -> [_ w313]
          tunnel: [w307 w308] -> w254
          tunnel: w261 -> [w307 w308]
          frame False {
          }
          frame True {
            n124 = call "Get Min.vi"("para_chn"=w313) -> ("function return"=→"CH1 Min":dbl)  [unwired: 9 in, 1 out]
            n125 = call "Get Max.vi"("para_chn"=w313) -> ("function return"=→"CH1 Max":dbl)  [unwired: 9 in, 1 out]
            n126 = call "Get Vpp.vi"("para_chn"=w313) -> ("function return"=→"CH1 Vpp":dbl)  [unwired: 9 in, 1 out]
            n127 = call "Get Freq.vi"("para_chn"=w313) -> ("function return"=→"CH1 Frequency":dbl)  [unwired: 9 in, 1 out]
          }
        }
        n128 = case shown="True" w243 {
          tunnel: w244 -> [_ w291]
          tunnel: [w285 w286] -> w253
          tunnel: w252 -> [w285 w286]
          frame False {
          }
          frame True {
            n129 = call "Get Min.vi"("para_chn"=w291) -> ("function return"=→"CH2 Min":dbl)  [unwired: 9 in, 1 out]
            n130 = call "Get Max.vi"("para_chn"=w291) -> ("function return"=→"CH2 Max":dbl)  [unwired: 9 in, 1 out]
            n131 = call "Get Vpp.vi"("para_chn"=w291) -> ("function return"=→"CH2 Vpp":dbl)  [unwired: 9 in, 1 out]
            n132 = call "Get Freq.vi"("para_chn"=w291) -> ("function return"=→"CH2 Frequency":dbl)  [unwired: 9 in, 1 out]
          }
        }
        n133 = Unbundle By Name(w240) -> ("Boolean <Is Exit>"=w267:bool)
        n134 = Select(t=w270, s=w267, f=w269) -> (s? t:f=w268:T2)
      }
      frame "Read IO" {
        w316 = FALSE  # Stop Loop?
        w317 = State."Wait for Event"  # Next State
        w323 = 16 ("front")
        w320 = 1 ("front")
        n135 = Unbundle By Name(w315) -> ("Device ID"=w314:dbl)
        n136 = call "Get IO In State.vi"("dev_id"=w314) -> ("function return"=w319:u32)  [unwired: 9 in, 1 out]
        "IO Read Return" <- w319
        n137 = And(x=w319, y=w323) -> (x .and. y?=w322:u32)
        n138 = And(x=w319, y=w320) -> (x .and. y?=w318:u32)
        n139 = Equal?(x=w318, y=w320) -> (x = y?=→"IO0":bool)
        n140 = Equal?(x=w322, y=w323) -> (x = y?=→"IO4":bool)
      }
      frame "Exit" {
        w331 = TRUE  # Stop Loop?
        w332 = State."Exit"  # (Value Not Used)
        # "#CodeNeeded - Add any required cleanup code here."
        # "The state value is not used here since this is the last iteration of the state machine loop."
        # "Exit - Exit the application."
        n141 = flat-sequence {
          tunnel: [w335] -> w329
          tunnel: w327 -> [w333]
          tunnel: [w333] -> w326
          tunnel: w329 -> [w342]
          tunnel: w326 -> [w340]
          frame #0 {
            w336 = i8 16  # IO Num
            w335 = i8 0  # en
            n142 = for {
              N: w336 -> [_]
              tunnel: w335 -> [w338]
              tunnel: w333 -> [w337]
              i -> [w339]
              n143 = call "IO Enable.vi"("enable"=w338, "channel"=w339, "dev_id"=w337) -> ()  [unwired: 8 in, 1 out]
            }
            n144 = Wait (ms)(milliseconds to wait=1000) -> ()  [unwired: 1 out]
          }
          frame #1 {
            w344 = i8 1  # channel
            w343 = i8 0  # channel
            n145 = call "DDS Output Enable.vi"("enable"=w342, "channel_index"=w343, "dev_id"=w340) -> ("error out"=w345:errorcluster)  [unwired: 8 in]
            n146 = call "DDS Output Enable.vi"("error in (no error)"=w345, "enable"=w342, "channel_index"=w344, "dev_id"=w340) -> ()  [unwired: 7 in, 1 out]
            n147 = Wait (ms)(milliseconds to wait=1000) -> ()  [unwired: 1 out]
          }
          frame #2 {
            n148 = call "Finish Dll.vi"() -> ()  [unwired: 10 in, 2 out]
          }
        }
        n149 = Unbundle By Name(w328) -> ("Device ID"=w327:dbl)
      }
    }
    n150 = Or(x=w7, y=w6) -> (x .or. y?=w8:bool)
  }
  n151 = call <vilib>:"Simple Error Handler.vi"("error in (no error)"=w2) -> ("error out"=w1:errorcluster)  [unwired: 4 in, 4 out]
  n152 = disable-structure shown="RUN_TIME_ENGINE==True" {
    disable-tunnel: w1 -> [_ _]
    frame condition #0 (active) {
    }
    frame condition #1 {
      # "Call Quit LabVIEW if running as a built application."
      n153 = Quit LabVIEW() -> ()  [unwired: 1 in]
    }
  }
